vi "PH_SystemInformation.set GUI Refs.vi"(0 "i ref in":refnum<vi>, 1 "Class":string, 2 "System Information GUI Refs":T1, 5 "error in (no error)":errorcluster) -> (14 "i ref out":refnum<vi>, 19 "error out":errorcluster)   [LabVIEW 2014, in "PH_SystemInformation.lvlib"]
doc: "By this VI the GUI refs are stored to own attributes."
uses:
  PH_SystemInformation.lvlib
  PH_SystemInformation.GUI Refs.ctl
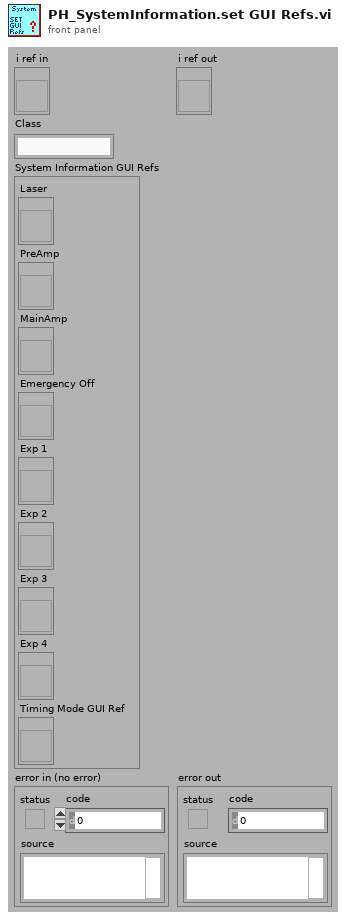
[diagram p1: front panel]
types:
  T1 = typedef "PH_SystemInformation.lvlib/PH_SystemInformation.GUI Refs.ctl" = cluster{"Laser":refnum<vi>, "PreAmp":refnum<vi>, "MainAmp":refnum<vi>, "Emergency Off":refnum<vi>, "Exp 1":refnum<vi>, "Exp 2":refnum<vi>, "Exp 3":refnum<vi>, "Exp 4":refnum<vi>, "Timing Mode GUI Ref":refnum<vi>}
  T2 = typedef "PH_SystemInformation.lvlib/PH_SystemInformation.i attribute.ctl" = cluster{"Laser Enabling":cluster{"GUI Ref":refnum<vi>, "Enabling State":T3}, "PreAmp Enabling":cluster{"GUI Ref":refnum<vi>, "Enabling State":T3}, "MainAmp Enabling":cluster{"GUI Ref":refnum<vi>, "Enabling State":T3}, "Emergency Off":cluster{"GUI Ref":refnum<vi>, "State":enum16{"no info", "off/false", "Alarm"}}, "Enabling Exp. 1":cluster{"GUI Ref":refnum<vi>, "Enabling State":T3}, "Enabling Exp. 2":cluster{"GUI Ref":refnum<vi>, "Enabling State":T3}, "Enabling Exp. 3":cluster{"GUI Ref":refnum<vi>, "Enabling State":T3}, "Enabling Exp. 4":cluster{"GUI Ref":refnum<vi>, "Enabling State":T3}, "Timing Mode":cluster{"GUI Ref":refnum<vi>, "PHELIX_Timing_Mode":enum32{"10 Hz", "0.5 Hz", "Shot"}}}
  T3 = typedef "PH_SystemInformation.lvlib/PH_SystemInformationEnabling State.ctl" = i32
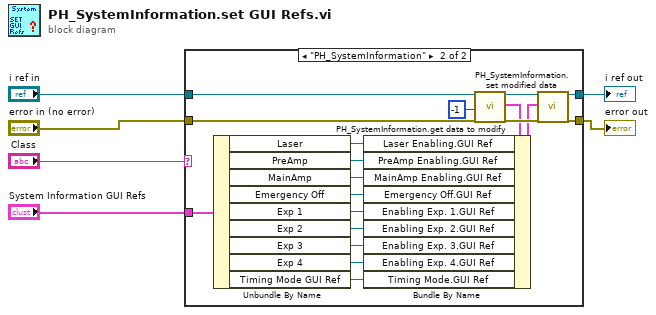
[diagram p0: block diagram]
diagram:
  n1 = case shown="\"PH_SystemInformation\"" "Class" {
    tunnel: "i ref in" -> [w8 w27]
    tunnel: "error in (no error)" -> [w7 w26]
    tunnel: "System Information GUI Refs" -> [_ w22]
    tunnel: [w8 w10] -> w3
    tunnel: [w7 w9] -> w2
    frame Default {
    }
    frame "PH_SystemInformation" {
      n2 = Unbundle By Name(w22) -> ("Laser"=w21:refnum<vi>, "PreAmp"=w20:refnum<vi>, "MainAmp"=w19:refnum<vi>, "Emergency Off"=w18:refnum<vi>, "Exp 1"=w17:refnum<vi>, "Exp 2"=w16:refnum<vi>, "Exp 3"=w15:refnum<vi>, "Exp 4"=w14:refnum<vi>, "Timing Mode GUI Ref"=w13:refnum<vi>)
      n3 = call "PH_SystemInformation.get data to modify.vi"("i ref in"=w27, "ms timeout (10000)"=-1, "error in (no error)"=w26) -> ("i ref out"=w23:refnum<vi>, "i attribute"=w24:T2, "error out"=w25:errorcluster)  [unwired: 13 in, 1 out]
      n4 = Bundle By Name(cluster=w24, "Laser Enabling.GUI Ref"=w21, "PreAmp Enabling.GUI Ref"=w20, "MainAmp Enabling.GUI Ref"=w19, "Emergency Off.GUI Ref"=w18, "Enabling Exp. 1.GUI Ref"=w17, "Enabling Exp. 2.GUI Ref"=w16, "Enabling Exp. 3.GUI Ref"=w15, "Enabling Exp. 4.GUI Ref"=w14, "Timing Mode.GUI Ref"=w13) -> (w12:T2)
      n5 = call "PH_SystemInformation.set modified data.vi"("i ref in"=w23, "i attribute"=w12, "error in (no error)"=w25) -> ("i ref out"=w10:refnum<vi>, "error out"=w9:errorcluster)  [unwired: 15 in]
    }
  }
  "i ref out" <- w3
  "error out" <- w2
